vi "Get Legend String.vi"(8 "error in (no error)":errorcluster caption="错误输入（无错误）", 10 "Legend Info":T1={"Name"="", "Percent"=0.0, "TxtColor"=0, "Hor Space"=0, "Ver Space"=5, "Color Segement"=[16448250, 0, 16736786, 1198079]}, 11 "Gradient PieChart 输入":refnum<class "Gradient PieChart.lvclass"> caption="DNL_LabVIEW Object in") -> (0 "error out":errorcluster caption="错误输出", 1 "TxtColor":u32(colorbox), 2 "Legend String":string, 3 "Gradient PieChart 输出":refnum<class "Gradient PieChart.lvclass"> caption="DNL_LabVIEW Object out")   [LabVIEW 2012, in "Gradient PieChart.lvclass"]
uses:
  Gradient PieChart.lvclass
  Legend Info.ctl
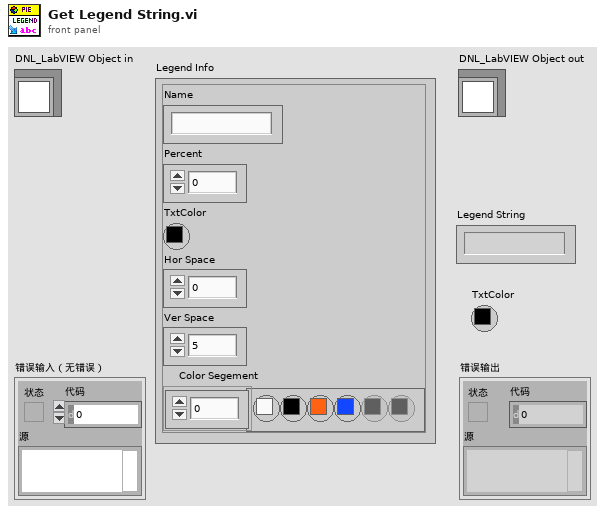
[diagram p1: front panel]
types:
  T1 = typedef "Gradient PieChart.lvclass/Legend Info.ctl" = cluster{"Name":string, "Percent":dbl, "TxtColor":u32, "Hor Space":i16, "Ver Space":i16, "Color Segement":u32[]}
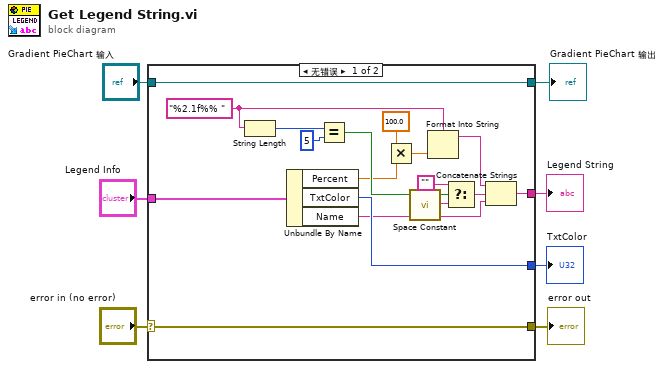
[diagram p0: block diagram]
diagram:
  n1 = case shown="无错误" "error in (no error)" {
    selector: "error in (no error)" -> [w23 w26]
    tunnel: [w23 w26] -> w6
    tunnel: [w24 w25] -> w4
    tunnel: "Gradient PieChart 输入" -> [w24 w25]
    tunnel: "Legend Info" -> [w22 _]
    tunnel: [w19 _] -> w2
    tunnel: [w21 _] -> w1
    frame No Error {
      w18 = "%2.1f%% " ("格式字符串")
      n2 = String Length(string=w18) -> (length=w17:i32)
      n3 = Unbundle By Name(w22) -> ("Percent"=w10:dbl, "TxtColor"=w21:u32, "Name"=w12:string)
      n4 = Equal?(x=w17, y=5) -> (x = y?=w15:bool)
      n5 = Multiply(x=100.0, y=w10) -> (x*y=w8:dbl)
      n6 = call <vilib>:"Space Constant.vi"() -> ("String"=w13:string)
      n7 = Format Into String(format string=w18, w8) -> (resulting string=w20:string)  [unwired: 2 in, 1 out]
      n8 = Select(t="", s=w15, f=w13) -> (s? t:f=w11:string)
      n9 = Concatenate Strings(w20, w11, w12) -> (w19:string)
    }
    frame Error {
    }
  }
  "error out" <- w6
  "Gradient PieChart 输出" <- w4
  "TxtColor" <- w1
  "Legend String" <- w2
